vi "Cleanup Client If Error.vi"(8 "error in":errorcluster, 10 "client name":string, 11 "project ref in":refnum<vi>) -> (0 "error out":errorcluster, 3 "project ref out":refnum<vi>)   [LabVIEW 2021, in "NI Measurement V2 Client Generator Runtime.lvlib"]
uses:
  NI Measurement V2 Client Generator Runtime.lvlib
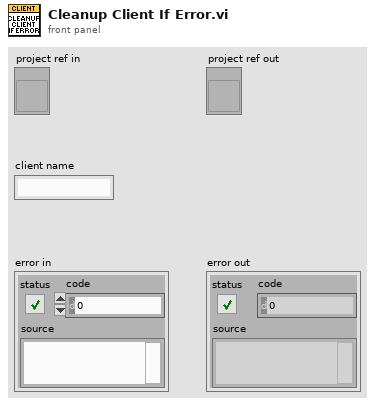
[diagram p1: front panel]
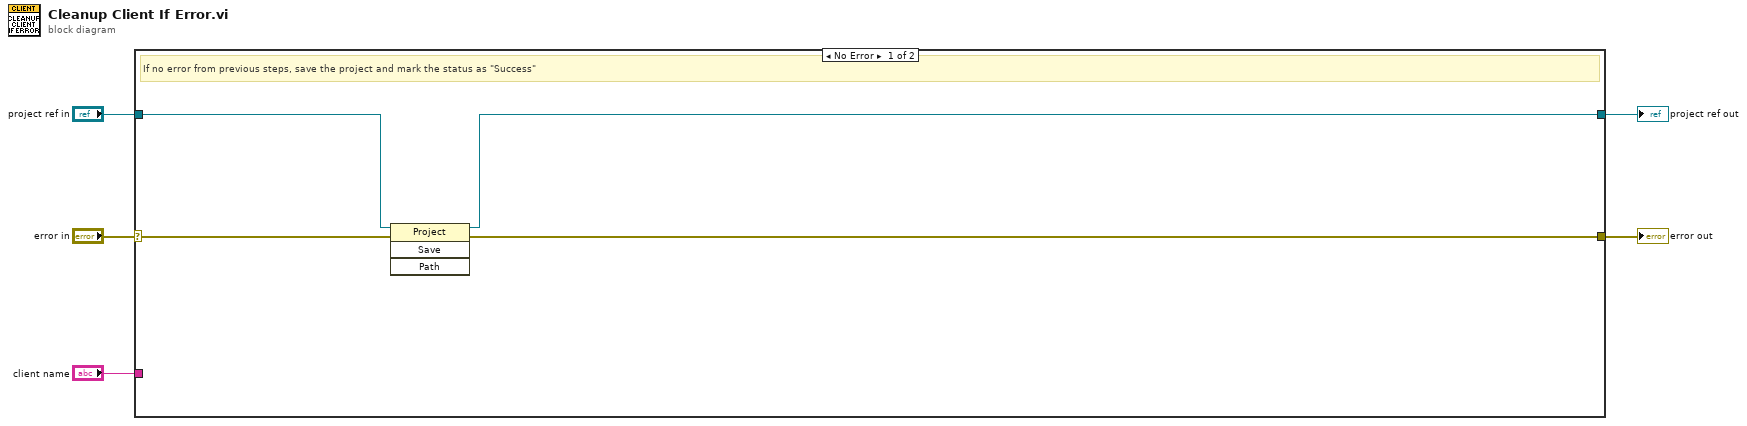
[diagram p0: block diagram]
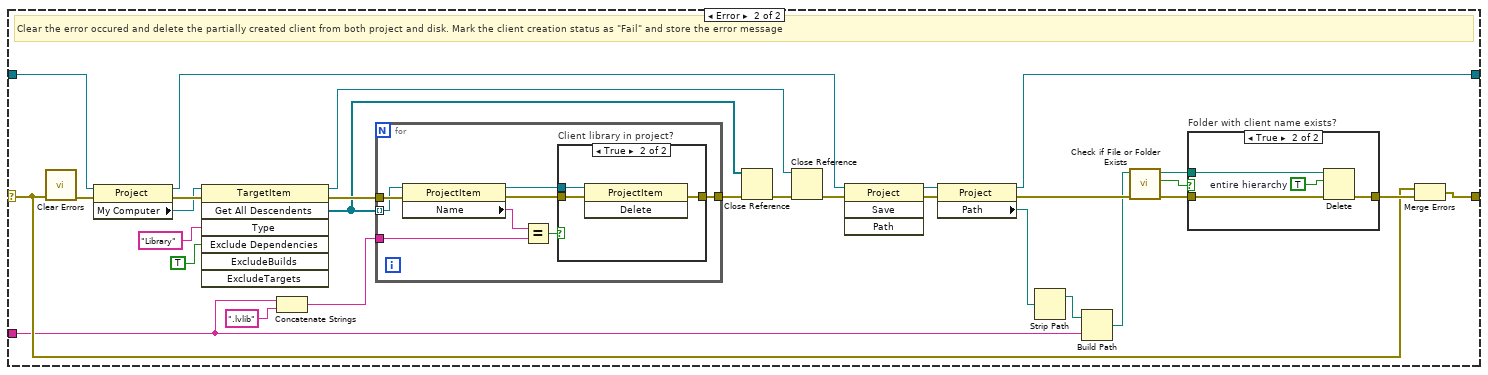
[diagram p2: hidden frame]
diagram:
  n1 = case shown="No Error" "error in" {
    selector: "error in" -> [w9 w12]
    tunnel: "project ref in" -> [w8 w38]
    tunnel: [w7 w27] -> w3
    tunnel: "client name" -> [_ w10]
    tunnel: [w6 w11] -> w1
    frame No Error {
      # "If no error from previous steps, save the project and mark the status as \"Success\""
      n2 = invoke class="Project" method="Save"(reference=w8, error in=w9) -> (reference out=w7:refnum<vi>, error out=w6:errorcluster)  [unwired: 2 in, 2 out]
    }
    frame Error {
      # "Clear the error occured and delete the partially created client from both project and disk. Mark the client creation status as \"Fail\" and store the error message"
      n3 = call <vilib>:"Clear Errors.vi"("error in (no error)"=w12) -> ("error out"=w31:errorcluster)  [unwired: 5 in, 1 out]
      n4 = property class="Project"(reference=w38, error in=w31) -> (reference out=w20:refnum<vi>, error out=w37:errorcluster, "My Computer"=w36:refnum<vi>)
      n5 = invoke class="TargetItem" method="Get All Descendents"(reference=w36, error in=w37, "Type"="Library", "Exclude Dependencies"=TRUE ("ExcludeDependencies")) -> (reference out=w29:refnum<vi>, error out=w33:errorcluster, "All Descendents"=w14:refnum<vi>[])  [unwired: 3 in, 4 out]
      n6 = Concatenate Strings(w10, ".lvlib" ("string")) -> (w17:string)
      n7 = for {
        tunnel: w33 -> [w51]
        tunnel: w14 -> [w50] mode=indexing
        tunnel: w17 -> [w48]
        tunnel: [w44] -> w32
        n8 = property class="ProjectItem"(reference=w50, error in=w51) -> (reference out=w47:refnum<vi>, error out=w45:errorcluster, "Name"=w49:string)
        n9 = Equal?(x=w49, y=w48) -> (x = y?=w46:bool)
        n10 = case "Client library in project?" shown="True" w46 {
          tunnel: w47 -> [_ w55]
          tunnel: w45 -> [w52 w54]
          tunnel: [w52 w53] -> w44
          frame False {
          }
          frame True {
            n11 = invoke class="ProjectItem" method="Delete"(reference=w55, error in=w54) -> (error out=w53:errorcluster)  [unwired: 1 in, 2 out]
          }
        }
      }
      n12 = Close Reference(reference=w14, error in (no error)=w32) -> (error out=w15:errorcluster)
      n13 = Close Reference(reference=w29, error in (no error)=w15) -> (error out=w30:errorcluster)
      n14 = invoke class="Project" method="Save"(reference=w20, error in=w30) -> (reference out=w19:refnum<vi>, error out=w21:errorcluster)  [unwired: 2 in, 2 out]
      n15 = property class="Project"(reference=w19, error in=w21) -> (reference out=w27:refnum<vi>, error out=w28:errorcluster, "Path"=w26:path)
      n16 = Strip Path(path=w26) -> (stripped path=w25:path)  [unwired: 1 out]
      n17 = Build Path(base path=w25, name or relative path=w10) -> (appended path=w24:path)
      n18 = call <vilib>:"Check if File or Folder Exists.vi"("error in (no error)"=w28, "path"=w24) -> ("error out"=w23:errorcluster, "file or folder exists?"=w16:bool, "dup path"=w22:path)  [unwired: 7 in]
      n19 = case "Folder with client name exists?" shown="True" w16 {
        tunnel: w23 -> [w39 w43]
        tunnel: [w39 w42] -> w13
        tunnel: w22 -> [_ w41]
        frame False {
        }
        frame True {
          w40 = TRUE  # entire hierarchy
          n20 = Delete(path (use dialog)=w41, entire hierarchy (F)=w40, error in=w43) -> (error out=w42:errorcluster)  [unwired: 2 in, 2 out]
        }
      }
      n21 = Merge Errors(w12, w13) -> (w11:errorcluster)
    }
  }
  "project ref out" <- w3
  "error out" <- w1
